vi "Pre Launch Init.vi"(11 "Report Generator_Tools in":refnum<class "Report Generator.lvclass">) -> (0 "error out":errorcluster, 3 "Report Generator_Tools out":refnum<class "Report Generator.lvclass">)   [LabVIEW 2019, in "Report Generator.lvlib" / "Report Generator.lvclass"]
uses:
  Library/Report Generator.lvclass
  builds/Base Software/Panels/Left Panel.lvlibp/Project/Left.lvclass
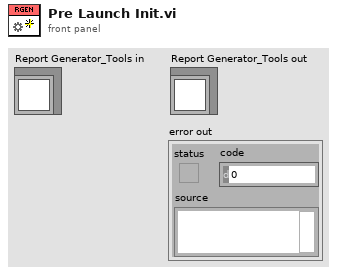
[diagram p1: front panel]
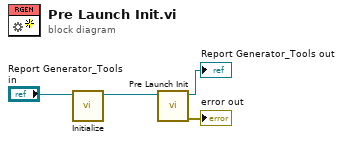
[diagram p0: block diagram]
diagram:
  n1 = call "Initialize.vi"("Report Generator in"="Report Generator_Tools in") -> ("Report Generator out"=w1:refnum<class "Report Generator.lvclass">)  [unwired: 9 in, 1 out]
  n2 = call-parent "Pre Launch Init.vi"("Engine_Tools in"=w1) -> ("error out"=→"error out":errorcluster, "Engine_Tools out"=→"Report Generator_Tools out":refnum<class "Report Generator.lvclass">)  [unwired: 9 in]
